vi "Shorten Cluster.vi"(3 "error in (no error)":errorcluster, 4 "Variant":variant, 5 "variable address in":string) -> (0 "error out":errorcluster, 1 "Variant":variant, 2 "variable address out":string)   [LabVIEW 2019, in "Logger.PGSQL.lvlib" / "Logger.PGSQL.lvclass"]
uses:
  Logger.PGSQL.lvclass
  <vilib>/Utility/Data Type/Type Definitions/Data Type.ctl
  <vilib>/Utility/Data Type/NI_Data Type.lvlib
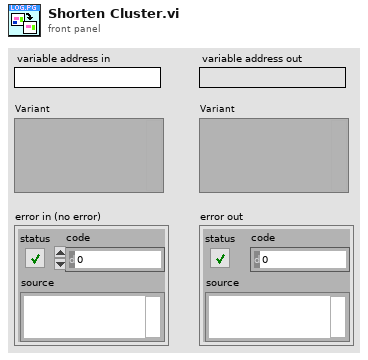
[diagram p1: front panel]
types:
  T1 = typedef "NI_Data Type.lvlib/Data Type.ctl" = enum8{"Invalid Type", "Void", "I8", "I16", "I32", "I64", "U8", "U16", "U32", "U64", "Single Float", "Double Float", "Extended Float", "Single Complex", "Double Complex", "Extended Complex", "Enum U8", "Enum U16", "Enum U32", "Enum U64", "Single Float With Unit", "Double Float With Unit", "Extended Float With Unit", "Single Complex with Unit", "Double Complex with Unit", "Extended Complex with Unit", "Boolean", "String", "Path", "Picture", "Tag", "Array", "Cluster", "Variant", "LV Variant", "Waveform", "Timestamp", "Digital Waveform", "Digital Data", "ExpressData", "Refnum", "External Data", "VI", "Poly VI", "LabVIEW Class Instance", "Fixed Point", "Set Collection", "Map Collection"}
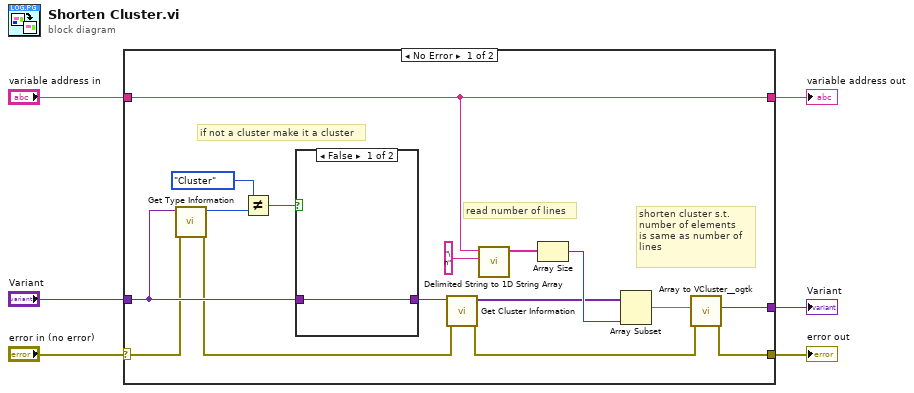
[diagram p0: block diagram]
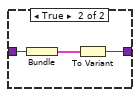
[diagram p2: hidden frame]
diagram:
  n1 = case shown="No Error" "error in (no error)" {
    selector: "error in (no error)" -> [w14 w28]
    tunnel: [w22 w28] -> w6
    tunnel: [w21 w29] -> w5
    tunnel: "variable address in" -> [w9 w27]
    tunnel: "Variant" -> [w17 w29]
    tunnel: [w9 w27] -> w1
    frame No Error {
      # "shorten cluster s.t.\nnumber of elements\nis same as number of \nlines"
      # "read number of lines"
      # "if not a cluster make it a cluster"
      n2 = call <vilib>:"Get Type Information.vi"("error in (no error)"=w14, "variant"=w17) -> ("error out"=w11:errorcluster, "type"=w20:T1)  [unwired: 5 in, 3 out]
      n3 = Not Equal?(x=Data_Type."Cluster" ("Type"), y=w20) -> (x != y?=w18:bool)
      n4 = case shown="False" w18 {
        tunnel: w17 -> [w23 w26]
        tunnel: [w23 w24] -> w13
        frame False {
        }
        frame True {
          n5 = Bundle("Variant"=w26) -> (w25:cluster{"Variant":variant})  [unwired: 1 in]
          n6 = To Variant(anything=w25) -> (Variant=w24:variant)
        }
      }
      n7 = call <vilib>:"Get Cluster Information.vi"("error in (no error)"=w11, "variant"=w13) -> ("error out"=w10:errorcluster, "cluster elements"=w12:variant[])  [unwired: 8 in]
      n8 = call <vilib>:"Delimited String to 1D String Array.vi"("delimiter"="\n", "delimited string"=w9) -> ("string array"=w7:string[])  [unwired: 9 in]
      n9 = Array Size(array=w7) -> (size(s)=w16:i32)
      n10 = Array Subset(array=w12, length=w16) -> (w15:variant[])  [unwired: 1 in]
      n11 = call <userlib>:"Array to VCluster__ogtk.vi"("error in (no error)"=w10, "Array"=w15) -> ("error out"=w22:errorcluster, "VCluster"=w21:variant)  [unwired: 8 in]
    }
    frame Error {
    }
  }
  "variable address out" <- w1
  "Variant" <- w5
  "error out" <- w6
